vi "stepperLeadScrewTest.vi"() -> ()   [LabVIEW 2019]
uses:
  <vilib>/ReMiSYS/ReMiSYS_myRIO-mini/SubVI/SYS/miniRef.ctl
panel:
  out "LC position now (cm)":dbl
  out "miniOut out":T1
  in  "miniOut in":T1
  in  "Set LC (cm)":dbl
  in  "Function":enum16{"init LC", "Set LC (cm)", "read LC"}(ring)
  out "ENC Counter (deg/s)":dbl
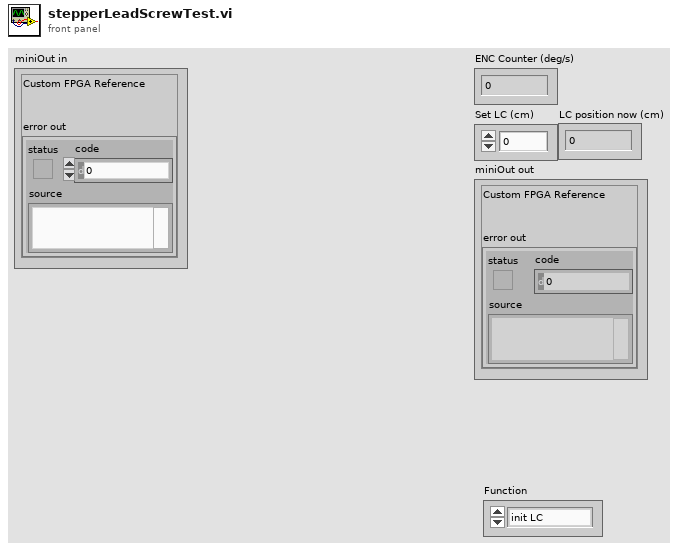
[diagram p1: front panel]
types:
  T1 = typedef "miniRef.ctl" = cluster{"Custom FPGA Reference":refnum<k20>, "error out":errorcluster}
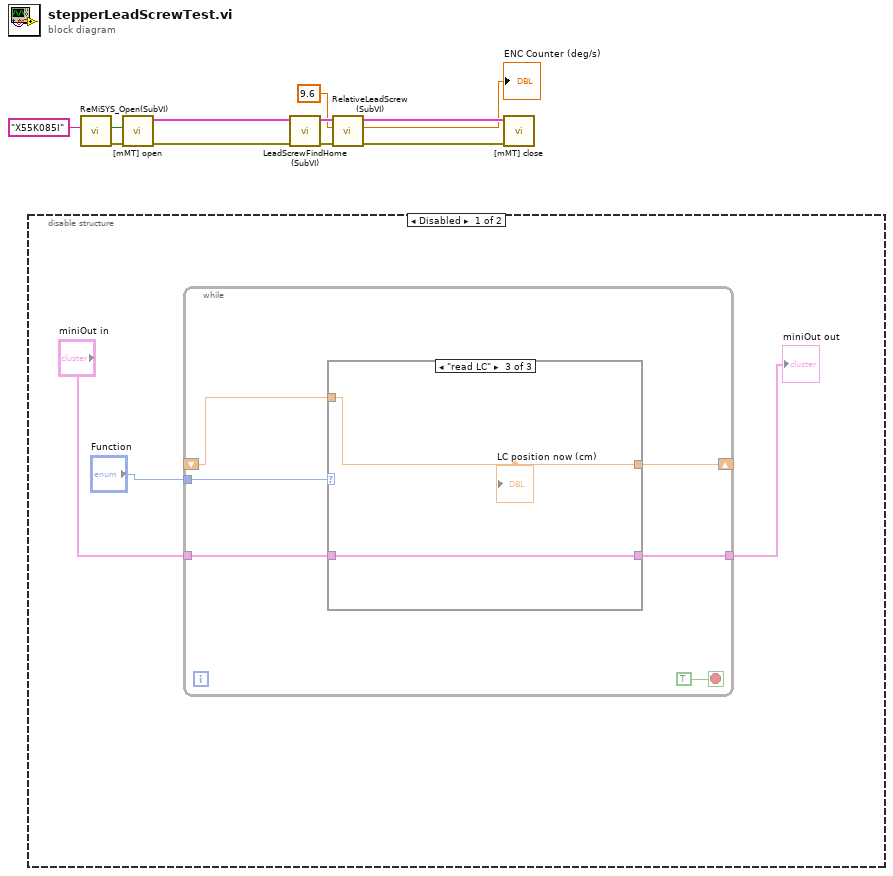
[diagram p0: block diagram]
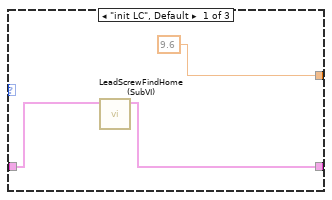
[diagram p2: hidden frame]
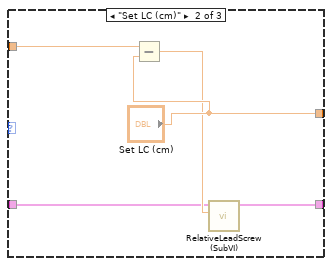
[diagram p3: hidden frame]
diagram:
  n1 = disable-structure shown="Disabled" {
    frame Disabled {
      n2 = while {
        tunnel: "Function" -> [w19]
        shift-right: [w18] -> _
        shift-left: _ -> [w17]
        tunnel: "miniOut in" -> [w16]
        tunnel: [w15] -> w12
        stop <- TRUE stop-if-true
        n3 = case shown="\"read LC\"" w19 {
          tunnel: [9.6 ("Distance (cm)") "Set LC (cm)" w30] -> w18
          tunnel: w17 -> [_ w27 w30]
          tunnel: w16 -> [w22 w25 w29]
          tunnel: [w21 w24 w29] -> w15
          frame "init LC", Default {
            n4 = call "LeadScrewFindHome (SubVI).vi"("miniOut in"=w22) -> ("miniOut out"=w21:T1)  [unwired: 7 in, 3 out]
          }
          frame "Set LC (cm)" {
            n5 = Subtract(x=w27, y="Set LC (cm)") -> (x-y=w26:dbl)
            n6 = call "RelativeLeadScrew (SubVI).vi"("Distance (cm)"=w26, "miniOut in"=w25) -> ("miniOut out"=w24:T1)  [unwired: 6 in, 3 out]
          }
          frame "read LC" {
            "LC position now (cm)" <- w30
          }
        }
      }
      "miniOut out" <- w12
    }
    frame Enabled {
    }
  }
  n7 = call <vilib>:"ReMiSYS_Open(SubVI).vi"("ReMiSYS Key"="X55K085I") -> ("error out"=w11:errorcluster, "Correct Key?"=w10:bool)  [unwired: 9 in]
  n8 = call <vilib>:"[mMT] open.vi"("error in"=w11, "Servo6,7"=w10) -> ("error out"=w6:errorcluster, "miniOut"=w5:T1)  [unwired: 7 in, 1 out]
  n9 = call "LeadScrewFindHome (SubVI).vi"("error in (no error)"=w6, "miniOut in"=w5) -> ("error out"=w3:errorcluster, "miniOut out"=w4:T1)  [unwired: 6 in, 2 out]
  n10 = call "RelativeLeadScrew (SubVI).vi"("error in (no error)"=w3, "Distance (cm)"=9.6, "miniOut in"=w4) -> ("error out"=w7:errorcluster, "ENC Counter (deg/s)"=→"ENC Counter (deg/s)":dbl, "miniOut out"=w8:T1)  [unwired: 5 in, 1 out]
  n11 = call <vilib>:"[mMT] close.vi"("error in (no error)"=w7, "miniOut in"=w8) -> ()  [unwired: 9 in, 1 out]
